vi "Error.Set-Change Error Info.vi"(6 "Std Code":T1 items=["No Error"=0, "Abort"=-2, "Misc"=-5000, "Fixture Error"=-5100, "File IO - General"=-5200, "FIle IO - Config Error"=-5201, "Instrument - General"=-5300, "Instrument - Serial Com"=-5301, "Instrument - Camera"=-5302, "Instrument - PS"=-5303, "Instrument - Oscilloscope"=-5304, "Instrument - Function Gen"=-5305, "Instrument - Load"=-5306, "Instrument - Meter"=-5307, "Instrument - Power Control"=-5308, "Instrument - Motion"=-5309, "Instrument - RF"=-5310, "System Exe"=-5400, "Image Processing"=-5500, "Communication"=-5600, "Script - Syntax Error"=-6000, "Script - Invalid Name or Param"=-6100, "Script - Timeout"=-6200, "Invalid Data"=-6300, "FW Update Error"=-6500], 7 "Append Details":bool=TRUE, 8 "error in":errorcluster, 9 "Description":string, 10 "Cust Code(0 = no change)":i32, 11 "Set Error":bool) -> (0 "error out":errorcluster)   [LabVIEW 2024, in "EQMF.lvlib" / "Errors.lvlib"]
uses:
  Errors.lvlib
  Error.Error Code List.ctl
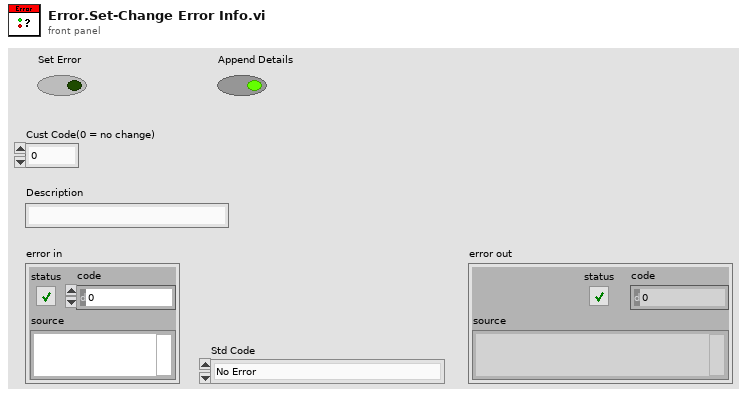
[diagram p1: front panel]
types:
  T1 = typedef "EQMF.lvlib/Errors.lvlib/Error.Error Code List.ctl" = i32
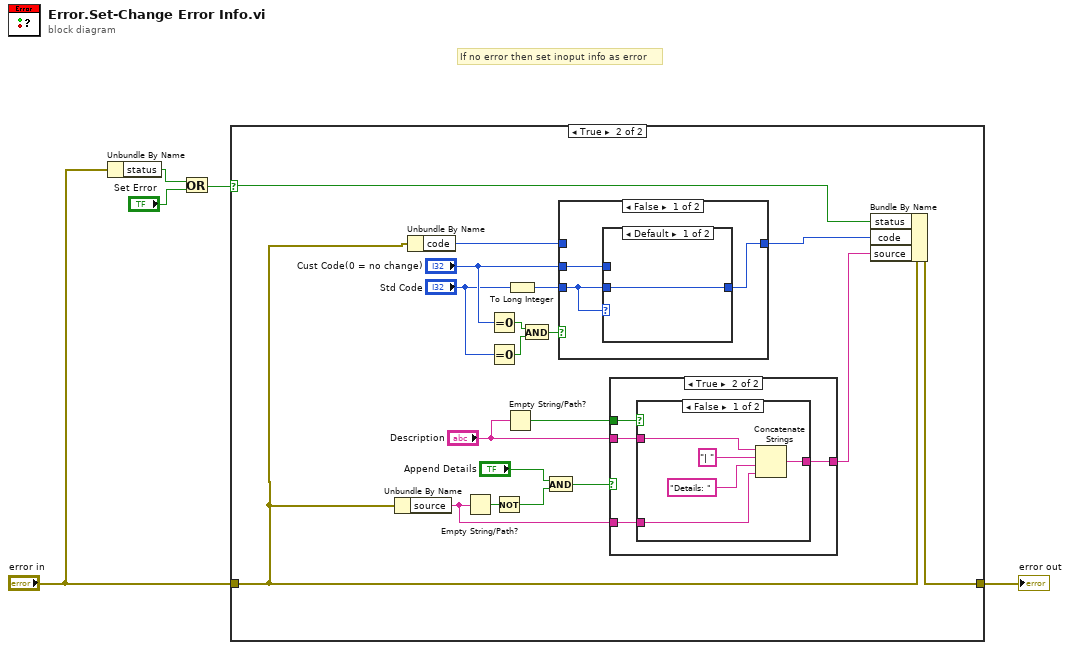
[diagram p0: block diagram]
diagram:
  # "If no error then set inoput info as error"
  n1 = Unbundle By Name("error in") -> ("status"=w4:bool)
  n2 = Or(x=w4, y="Set Error") -> (x .or. y?=w1:bool)
  n3 = case shown="True" w1 {
    selector: w1 -> [_ w7]
    tunnel: [w6 w25] -> w5
    tunnel: "error in" -> [w6 w8]
    frame False {
    }
    frame True {
      n4 = Unbundle By Name(w8) -> ("source"=w17:string)
      n5 = Unbundle By Name(w8) -> ("code"=w18:i32)
      n6 = Empty String/Path?(string/path=w17) -> (empty?=w24:bool)
      n7 = Equal To 0?(x="Cust Code(0 = no change)") -> (x = 0?=w13:bool)
      n8 = Equal To 0?(x="Std Code") -> (x = 0?=w12:bool)
      n9 = Not(x=w24) -> (.not. x?=w22:bool)
      n10 = Empty String/Path?(string/path="Description") -> (empty?=w15:bool)
      n11 = To Long Integer(number="Std Code") -> (32bit integer=w9:T1)
      n12 = And(x=w13, y=w12) -> (x .and. y?=w14:bool)
      n13 = And(x="Append Details", y=w22) -> (x .and. y?=w20:bool)
      n14 = case shown="False" w14 {
        tunnel: [w28 w31] -> w19
        tunnel: w18 -> [_ w31]
        tunnel: "Cust Code(0 = no change)" -> [w27 _]
        tunnel: w9 -> [w26 _]
        frame False {
          n15 = case shown="Default" w26 {
            tunnel: w27 -> [_ w30]
            tunnel: [w29 w30] -> w28
            tunnel: w26 -> [w29 _]
            frame Default {
            }
            frame 0 {
            }
          }
        }
        frame True {
        }
      }
      n16 = case shown="True" w20 {
        tunnel: "Description" -> [w32 w41]
        tunnel: [w34 w40] -> w21
        tunnel: w17 -> [w33 w39]
        tunnel: w15 -> [w35 w38]
        frame False {
          n17 = case shown="False" w35 {
            tunnel: [w36 w37] -> w34
            tunnel: w33 -> [_ w37]
            tunnel: w32 -> [w36 _]
            frame False {
            }
            frame True {
            }
          }
        }
        frame True {
          n18 = case shown="False" w38 {
            tunnel: w41 -> [w45 _]
            tunnel: [w44 w47] -> w40
            tunnel: w39 -> [w43 w47]
            frame False {
              n19 = Concatenate Strings(w45, "| ", "Details: ", w43) -> (w44:string)
            }
            frame True {
            }
          }
        }
      }
      n20 = Bundle By Name(cluster=w8, "status"=w7, "code"=w19, "source"=w21) -> (w25:errorcluster)
    }
  }
  "error out" <- w5
